vi "Priority Enqueue.vi"(6 "timeout in ms (-1)":i32=-1, 8 "error in (no error)":errorcluster, 9 "data":T1, 10 "priority":u32, 11 "Bounded Priority Queue in":refnum<class "Bounded Priority Queue.lvclass">) -> (0 "error out":errorcluster, 1 "timed out?":bool, 3 "Bounded Priority Queue out":refnum<class "Bounded Priority Queue.lvclass">)   [LabVIEW 2011, in "Bounded Priority Queue.lvclass"]
uses:
  Bounded Priority Queue.lvclass
  Data.ctl
  Bounded Priority Queue.lvclass/Bounded Priority Queue.ctl
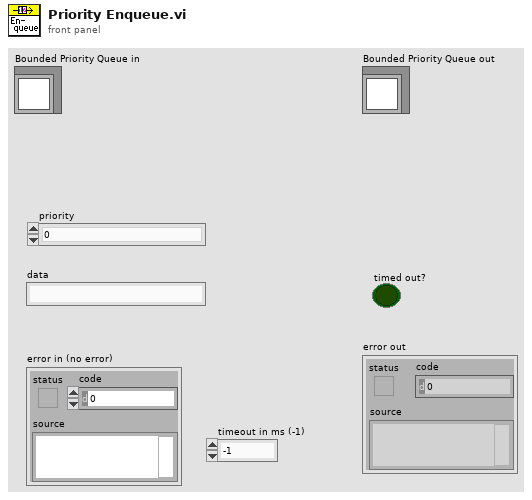
[diagram p1: front panel]
types:
  T1 = typedef "Bounded Priority Queue.lvclass/Data.ctl" = string
  T2 = typedef "Priority Queue.lvclass/DVR Contents.ctl" = cluster{"# Waiting":u32, "Buffers":refnum<queue>[], "How Many Priorities":u32, "Bounding":refnum<queue>}
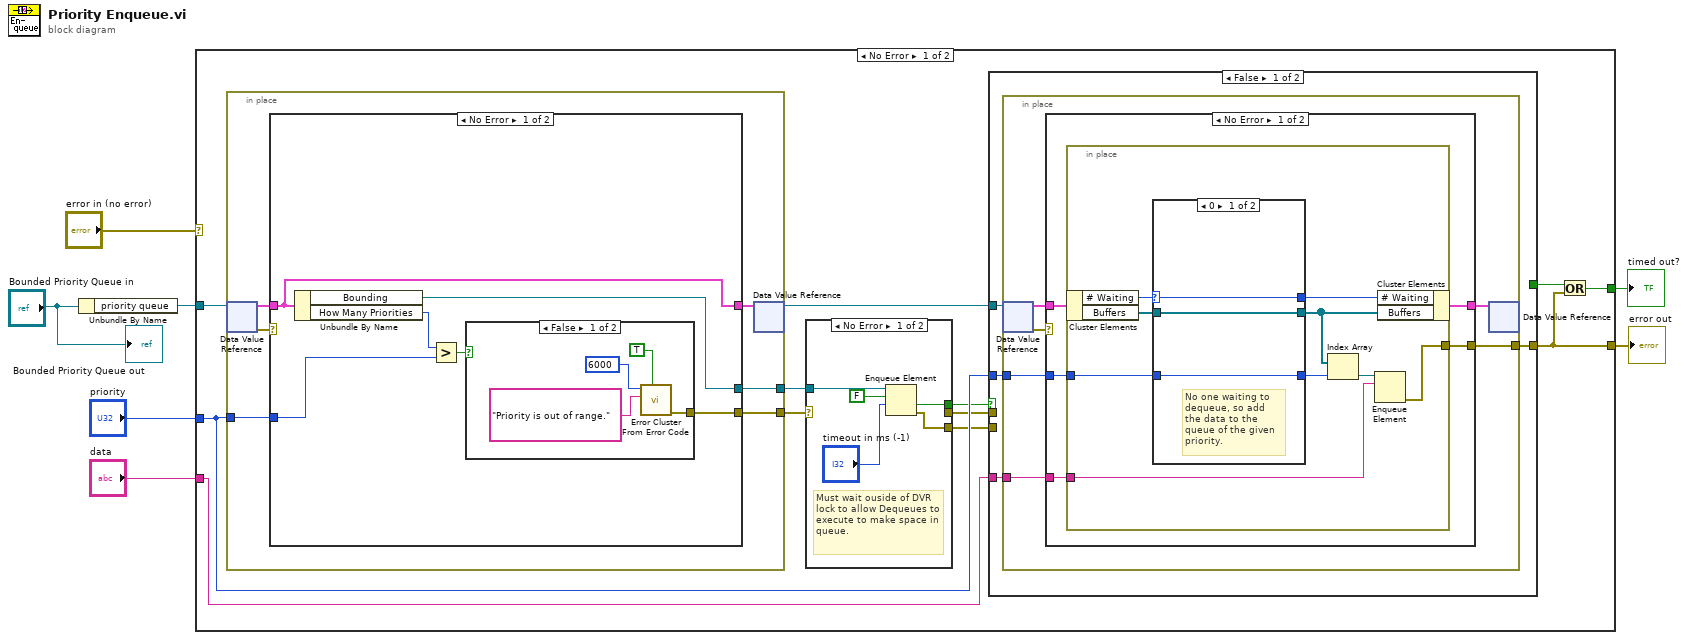
[diagram p0: block diagram]
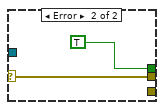
[diagram p2: hidden frame]
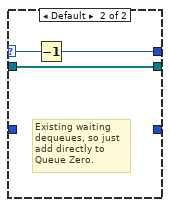
[diagram p3: hidden frame]
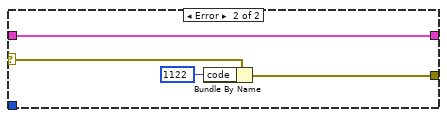
[diagram p4: hidden frame]
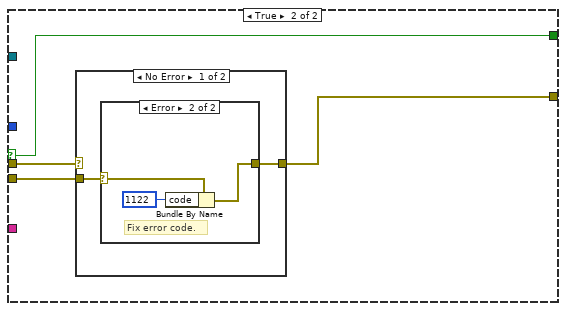
[diagram p5: hidden frame]
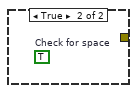
[diagram p8: hidden frame]
diagram:
  n1 = Unbundle By Name("Bounded Priority Queue in") -> ("priority queue"=w3:refnum<data-value>)
  n2 = case shown="No Error" "error in (no error)" {
    selector: "error in (no error)" -> [_ w90]
    tunnel: [w10 w90] -> w6
    tunnel: w3 -> [w19 _]
    tunnel: "data" -> [w17 _]
    tunnel: "priority" -> [w16 _]
    tunnel: [w9 _] -> w1
    frame No Error {
      n3 = in-place {
        in-place-border: [w76] -> w15
        in-place-border: w16 -> [w73]
        in-place-border: [w72] -> w14
        n4 = in-place-dvr #1(w19) -> (w74:T2, w77:errorcluster)
        n5 = case shown="No Error" w77 {
          selector: w77 -> [_ w89]
          tunnel: [w82 w89] -> w76
          tunnel: [w79 w88] -> w75
          tunnel: w74 -> [w79 w88]
          tunnel: w73 -> [w83 _]
          tunnel: [w78 _] -> w72
          frame No Error {
            n6 = Unbundle By Name(w79) -> ("Bounding"=w78:refnum<queue>, "How Many Priorities"=w80:u32)
            n7 = Greater?(x=w80, y=w83) -> (0:w81:bool)
            n8 = case shown="False" w81 {
              tunnel: [w84 _] -> w82
              frame False {
                n9 = call <vilib>:"Error Cluster From Error Code.vi"("show call chain? (False)"=TRUE, "error message (\"\")"="Priority is out of range." ("error message (\"\")"), "error code (0)"=6000) -> ("error out"=w84:errorcluster)  [unwired: 6 in]
              }
              frame True {
                (unwired) TRUE  # Check for space
              }
            }
          }
          frame Error {
          }
        }
        n10 = in-place-dvr #1(w75) -> (w18:refnum<data-value>)  [unwired: 1 out]
      }
      n11 = case shown="No Error" w15 {
        selector: w15 -> [_ w26]
        tunnel: w14 -> [w24 _]
        tunnel: [_ w26] -> w12
        tunnel: [w21 TRUE ("timed out?")] -> w13
        tunnel: [w20 _] -> w8
        frame No Error {
          # "Must wait ouside of DVR lock to allow Dequeues to execute to make space in queue."
          n12 = Enqueue Element(queue=w24, element=FALSE, timeout in ms (-1)="timeout in ms (-1)") -> (timed out?=w21:bool, error out=w20:errorcluster)  [unwired: 1 in, 1 out]
        }
        frame Error {
        }
      }
      n13 = case shown="False" w13 {
        selector: w13 -> [_ w64]
        tunnel: w18 -> [w30 _]
        tunnel: [w29 w61] -> w10
        tunnel: w16 -> [w28 _]
        tunnel: w17 -> [w27 _]
        tunnel: w12 -> [_ w62]
        tunnel: [_ w64] -> w11
        tunnel: w8 -> [_ w63]
        frame False {
          n14 = in-place {
            in-place-border: [w35] -> w29
            in-place-border: w27 -> [w32]
            in-place-border: w28 -> [w31]
            n15 = in-place-dvr #2(w30) -> (w33:T2, w36:errorcluster)
            n16 = case shown="No Error" w36 {
              selector: w36 -> [_ w59]
              tunnel: [w37 w58] -> w35
              tunnel: [w39 w60] -> w34
              tunnel: w33 -> [w41 w60]
              tunnel: w32 -> [w40 _]
              tunnel: w31 -> [w38 _]
              frame No Error {
                n17 = in-place {
                  in-place-border: w40 -> [w49]
                  in-place-border: w38 -> [w44]
                  in-place-border: [w45] -> w37
                  n18 = in-place-cluster #3(w41) -> ("# Waiting"=w47:u32, "Buffers"=w50:refnum<queue>[])
                  n19 = case shown="0" w47 {
                    selector: w47 -> [w53 w55]
                    tunnel: w50 -> [w52 w56]
                    tunnel: [w52 w56] -> w48
                    tunnel: [w53 w54] -> w46
                    tunnel: w44 -> [w51 _]
                    tunnel: [w51 _] -> w42
                    frame 0 {
                      # "No one waiting to\ndequeue, so add\nthe data to the \nqueue of the given\npriority."
                    }
                    frame Default {
                      # "Existing waiting\ndequeues, so just\nadd directly to\nQueue Zero."
                      n20 = Decrement(x=w55) -> (x-1=w54:u32)
                    }
                  }
                  n21 = Index Array(array=w48, index=w42) -> (element=w43:refnum<queue>)
                  n22 = Enqueue Element(queue=w43, element=w49) -> (error out=w45:errorcluster)  [unwired: 2 in, 2 out]
                  n23 = in-place-cluster #3("# Waiting"=w46, "Buffers"=w48) -> (w39:T2)
                }
              }
              frame Error {
                n24 = Bundle By Name(cluster=w59, "code"=1122) -> (w58:errorcluster)
              }
            }
            n25 = in-place-dvr #2(w34) -> ()  [unwired: 2 out]
          }
        }
        frame True {
          n26 = case shown="No Error" w62 {
            selector: w62 -> [_ w71]
            tunnel: w63 -> [w66 _]
            tunnel: [w65 w71] -> w61
            frame No Error {
              n27 = case shown="Error" w66 {
                selector: w66 -> [w67 w69]
                tunnel: [w67 w68] -> w65
                frame No Error {
                }
                frame Error {
                  # "Fix error code."
                  n28 = Bundle By Name(cluster=w69, "code"=1122) -> (w68:errorcluster)
                }
              }
            }
            frame Error {
            }
          }
        }
      }
      n29 = Or(x=w11, y=w10) -> (x .or. y?=w9:bool)
    }
    frame Error {
    }
  }
  "error out" <- w6
  "timed out?" <- w1
  "Bounded Priority Queue out" <- "Bounded Priority Queue in"
